vi "Main.vi"() -> ()   [LabVIEW 2020, in "LV Client.lvclass"]
uses:
  LV Client.lvclass
  LV Client.lvclass/LV Client.ctl
  _Main Async.vi
panel:
  in  "Server TCP Port":u16=4763
  in  "Server Address":string="127.0.0.1"
  # "Make sure the above values match the server address and port and then run this VI. A new client instance is created each time this VI is run."
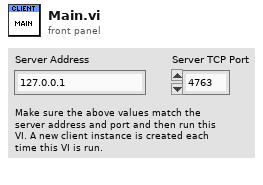
[diagram p1: front panel]
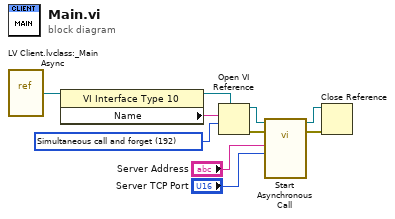
[diagram p0: block diagram]
diagram:
  w5 = 192 items=["Record modifications"=1, "Open templates for editing"=2, "Prompt user to save"=4, "Prepare for reentrant run"=8, "Prompt to find missing subVIs"=16, "Hide loading dialog box"=32, "Enable simultaneous calls"=64, "Prepare to call and forget"=128, "Simultaneous call and forget"=192, "Prepare to call and collect"=256, "Simultaneous call and collect"=320]
  n1 = vi-ref "LV Client.lvclass:_Main Async.vi"() -> (w3:refnum<vi>)
  n2 = property class="VI Interface Type 10"(reference=w3) -> (reference out=w6:refnum<vi>, "Name"=w4:string)  [unwired: 1 in, 1 out]
  n3 = Open VI Reference(type specifier VI Refnum (for type only)=w6, vi path=w4, options=w5) -> (vi reference=w8:refnum<vi>, error out=w7:errorcluster)  [unwired: 3 in]
  n4 = call-by-ref "Start Asynchronous Call"(reference=w8, error in=w7, "Server TCP Port"="Server TCP Port", "Server Address"="Server Address") -> (reference out=w10:refnum<vi>, error out=w9:errorcluster)  [unwired: 10 in]
  n5 = Close Reference(reference=w10, error in (no error)=w9) -> ()  [unwired: 1 out]
